vi "Test timer.vi"() -> ()   [LabVIEW 2012]
panel:
  out "Array":dbl[](array[numeric])
  in  "Target Time Sec":dbl=5.0
  in  "Pause":bool
  out "Remaining Time":dbl
  out "Time Expired":bool
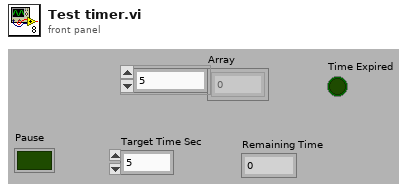
[diagram p1: front panel]
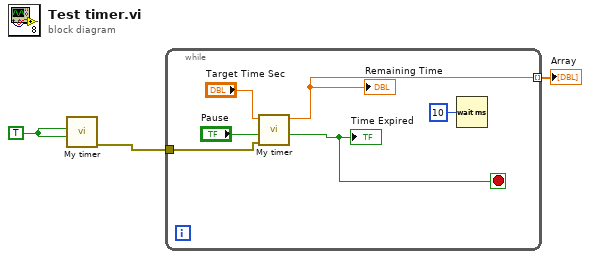
[diagram p0: block diagram]
diagram:
  w2 = TRUE ("Reset")
  n1 = call "My timer.vi"("Reset"=w2, "Pause"=w2) -> ("error out"=w3:errorcluster)  [unwired: 2 in, 6 out]
  n2 = while {
    tunnel: w3 -> [w6]
    tunnel: [w4] -> w1 mode=indexing
    stop <- w8 stop-if-true
    n3 = call "My timer.vi"("Target Time Sec"="Target Time Sec", "Pause"="Pause", "error in (no error)"=w6) -> ("Remaining Time"=w4:dbl, "Time Expired"=w8:bool)  [unwired: 1 in, 5 out]
    "Time Expired" <- w8
    "Remaining Time" <- w4
    n4 = Wait (ms)(milliseconds to wait=u32 10) -> ()  [unwired: 1 out]
  }
  "Array" <- w1
